vi "haslength.vi"(11 "port":refnum<visa-resource-name>) -> (3 "haslength":bool)   [LabVIEW 2012]
uses:
  <vilib>/Instr/_visa.llb/VISA Configure Serial Port (Instr).vi
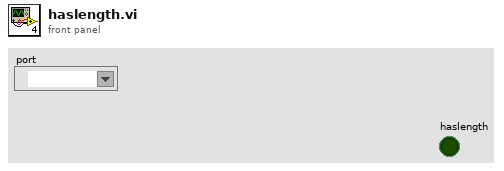
[diagram p1: front panel]
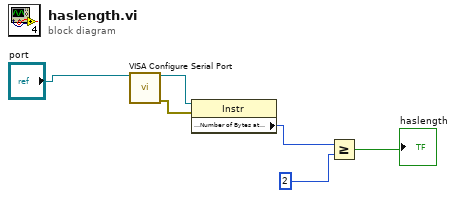
[diagram p0: block diagram]
diagram:
  n1 = call-poly "VISA Configure Serial Port"("VISA resource name"="port") -> ("VISA resource name out"=w1:refnum<visa-resource-name>, "error out"=w2:errorcluster)  [unwired: 13 in]
  n2 = property class="Instr"(reference=w1, error in=w2) -> ("Serial Settings:Number of Bytes at Serial Port"=w5:u32)  [unwired: 2 out]
  n3 = Greater Or Equal?(x=w5, y=2) -> (x >= y?=→"haslength":bool)
